vi "header.vi"(0 "Signals":dbl[](array[numeric]), 2 "标准差 V":dbl=0.02 format="%.2p", 3 "采样数 k":dbl=3000.0, 4 "Lower Cut-Off":dbl=280000.0, 8 "采样率 MHz":dbl=50.0, 9 "f_c kHz":dbl=150.0, 10 "A_c V":dbl=1.0, 11 "k_f kHz/V":dbl=50.0) -> (5 "解调复原的基带信号":waveform(dbl)(graph), 6 "已调信号频域波形观测":dynamicdata(graph), 7 "信号时域波形观测":dynamicdata(graph))   [LabVIEW 2020]
uses:
  <vilib>/express/express shared/transition.llb/Dynamic To Waveform Array.vi
  <vilib>/express/express arith-compare/Formula/Block/exnFormulaBlock how many pts in the wave.vi
  <vilib>/express/express shared/ex_Modify Signal Name.vi
  <vilib>/express/express shared/transition.llb/Waveform Array To Dynamic.vi
  <vilib>/express/express analysis/Spectral/Block/exnSpectralBlock spectral measurements peak poly.vi
  <vilib>/express/express analysis/Spectral/Block/exnSpectralBlock spectral measurements peak DDT.vi
  <vilib>/express/express arith-compare/Formula/XNode/ExpressFormulaBlockNode.xnode
  <vilib>/express/express analysis/Spectral/XNode/ExpressSpectralMeasurementsBlockNode.xnode
  <vilib>/measure/NI_MABase.lvlib
  <vilib>/Analysis/NI_AALPro.lvlib
panel:
  out "f_c Hz":dbl
  out "采样数":dbl
  out "采样率 Hz":dbl
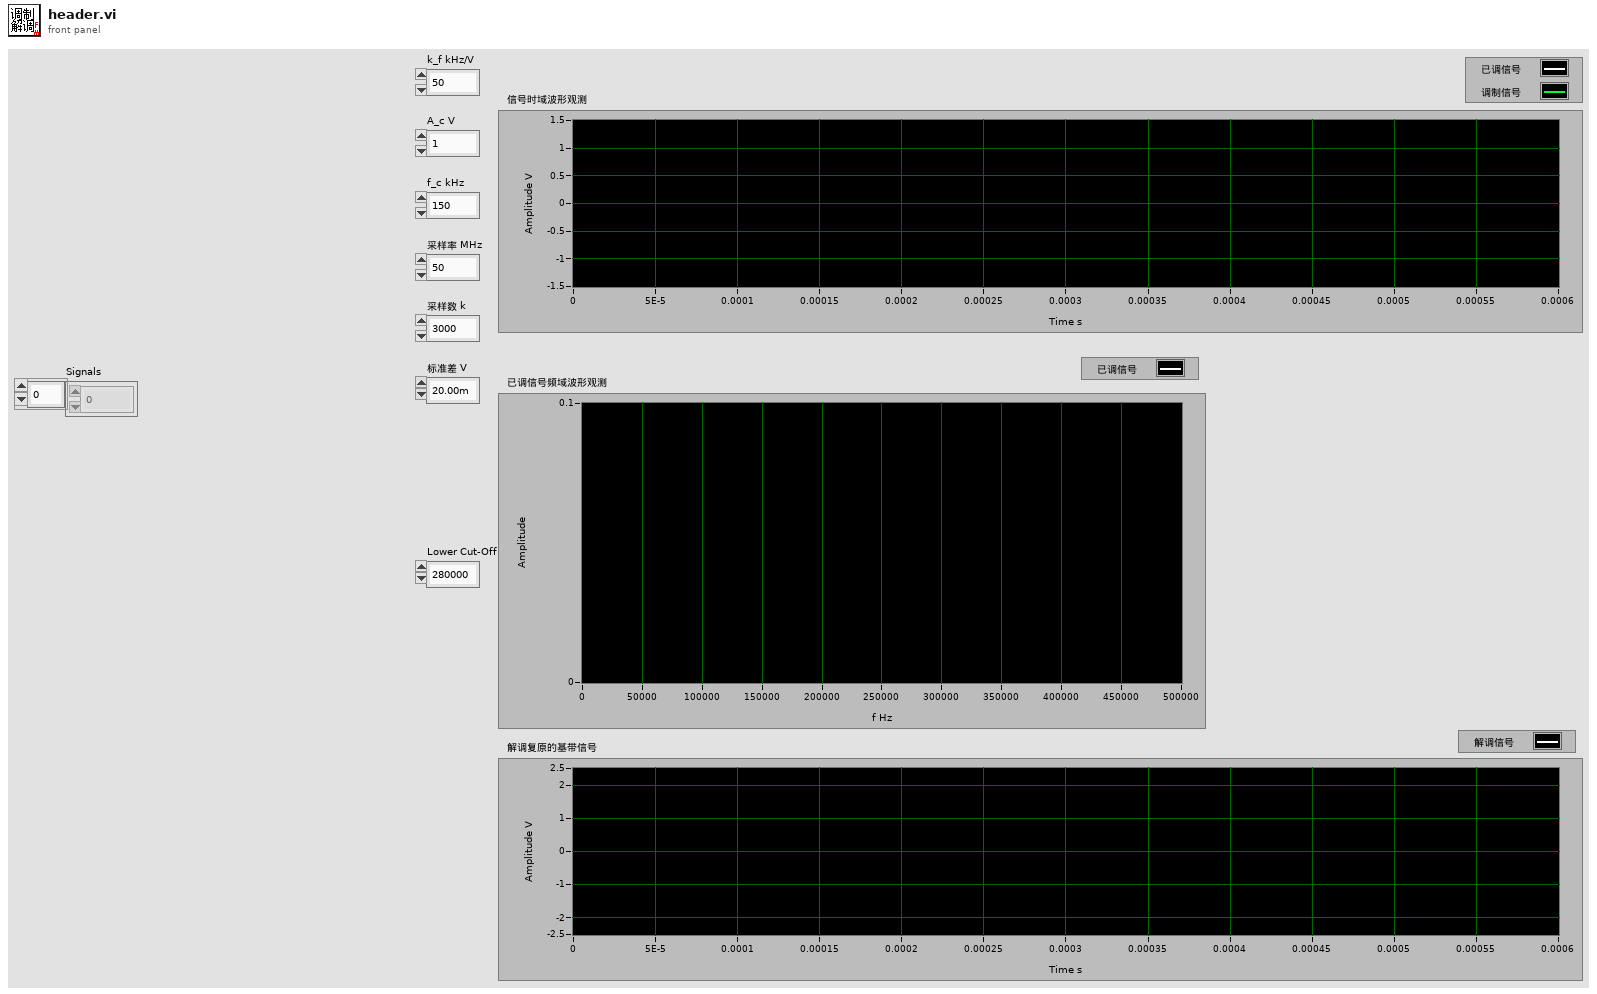
[diagram p1: front panel]
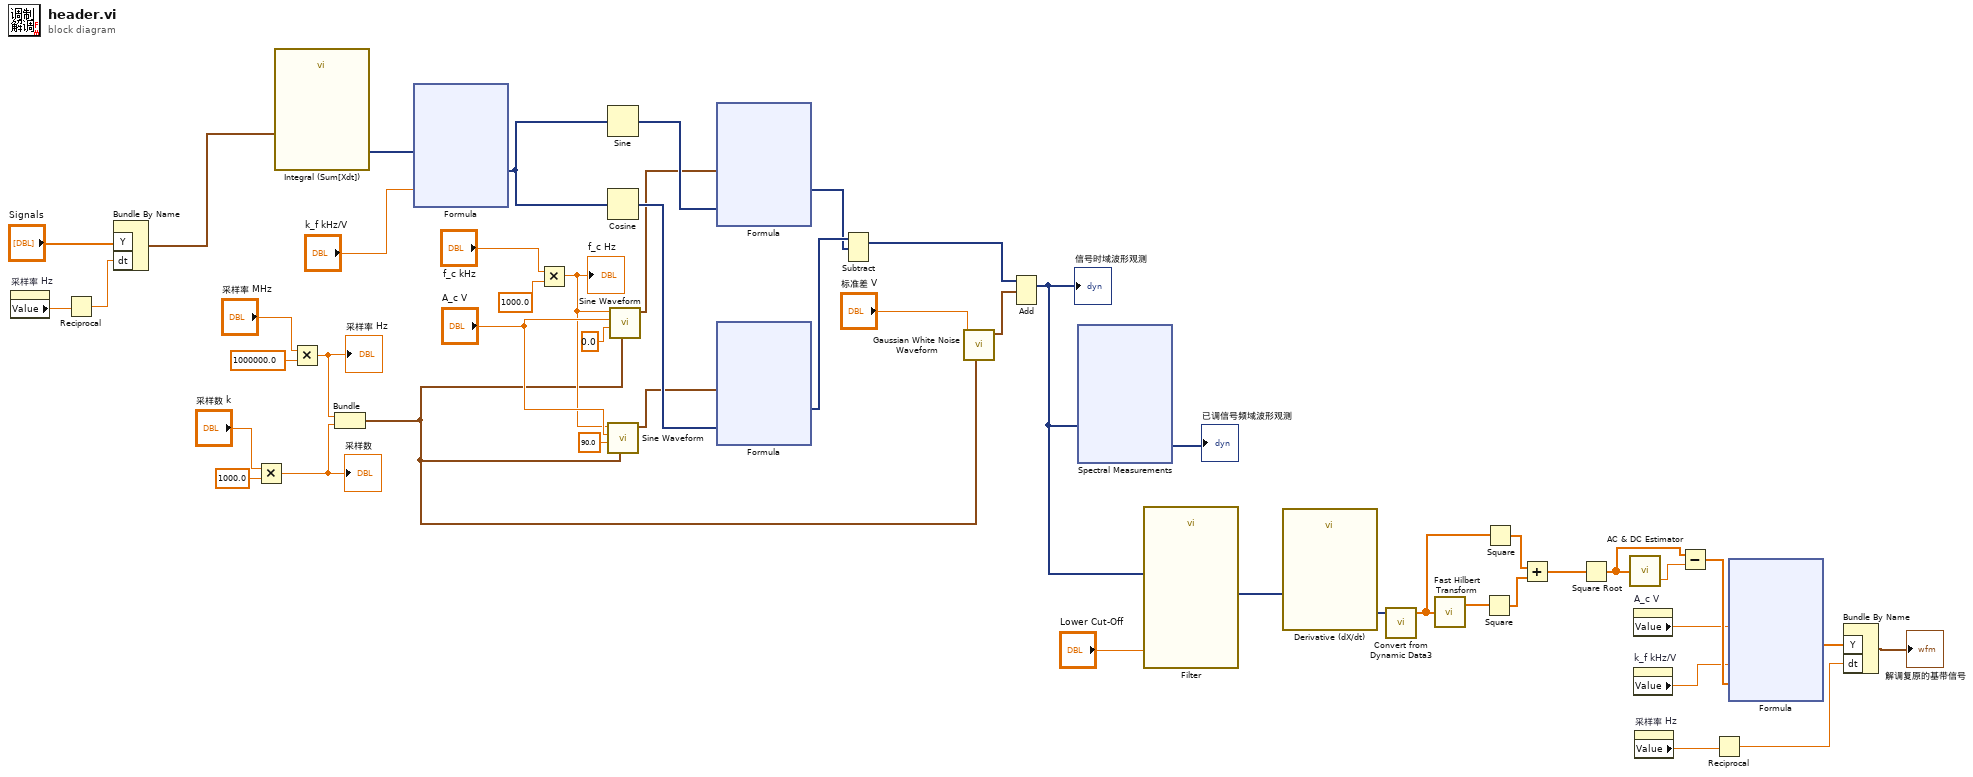
[diagram p0: block diagram]
diagram:
  n1 = property on="采样率 Hz" class="DigNum (strict)"() -> ("Value"=w2:dbl)  [unwired: 2 in, 2 out]
  n2 = Reciprocal(x=w2) -> (1/x=w5:dbl)
  n3 = Bundle By Name("Y"="Signals", "dt"=w5) -> (w3:waveform(dbl))  [unwired: 1 in]
  n4 = Multiply(x="采样数 k", y=1000.0) -> (x*y=w35:dbl)
  "采样数" <- w35
  n5 = call "Integral (Sum[Xdt])"("Signals"=w3) -> ("Result"=w25:dynamicdata)  [unwired: 5 in, 1 out]
  n6 = Multiply(x="采样率 MHz", y=1000000.0) -> (x*y=w38:dbl)
  "采样率 Hz" <- w38
  n7 = Bundle(w38, w35) -> (w23:cluster{dbl, dbl})  [unwired: 1 in]
  n8 = xnode "Formula"("积分后的信号"=w25, "k_f"="k_f kHz/V") -> ("Result"=w47:dynamicdata)  [unwired: 1 in, 1 out]
  n9 = Multiply(x="f_c kHz", y=1000.0) -> (x*y=w41:dbl)
  "f_c Hz" <- w41
  n10 = Sine(x=w47) -> (sin(x)=w33:dynamicdata)
  n11 = Cosine(x=w47) -> (cos(x)=w34:dynamicdata)
  n12 = call <vilib>:"Sine Waveform.vi"("sampling info"=w23, "phase"=90.0, "amplitude"="A_c V", "frequency"=w41) -> ("signal out"=w31:waveform(dbl))  [unwired: 6 in, 1 out]
  n13 = call <vilib>:"Sine Waveform.vi"("sampling info"=w23, "phase"=0.0, "amplitude"="A_c V", "frequency"=w41) -> ("signal out"=w32:waveform(dbl))  [unwired: 6 in, 1 out]
  n14 = xnode "Formula"("sin载波"=w32, "sin相偏"=w33) -> ("Result"=w29:dynamicdata)  [unwired: 1 in, 1 out]
  n15 = xnode "Formula"("cos载波"=w31, "cos相偏"=w34) -> ("Result"=w30:dynamicdata)  [unwired: 1 in, 1 out]
  n16 = Subtract(1:w29, 2:w30) -> (0:w27:dynamicdata)  [unwired: 1 in, 1 out]
  n17 = call <vilib>:"Gaussian White Noise Waveform.vi"("sampling info"=w23, "standard deviation"="标准差 V") -> ("signal out"=w26:waveform(dbl))  [unwired: 8 in, 1 out]
  n18 = Add(1:w26, 2:w27) -> (0:w1:dynamicdata)  [unwired: 1 in, 1 out]
  "信号时域波形观测" <- w1
  n19 = xnode "Spectral Measurements"("Signals"=w1) -> ("FFT - (Peak)"=→"已调信号频域波形观测":dynamicdata)  [unwired: 1 in, 2 out]
  n20 = call "Filter"("Lower Cut-Off"="Lower Cut-Off", "Signal"=w1) -> ("Filtered Signal"=w7:dynamicdata)  [unwired: 8 in, 1 out]
  n21 = call "Derivative (dX/dt)"("Signals"=w7) -> ("Result"=w17:dynamicdata)  [unwired: 5 in, 1 out]
  n22 = call "Convert from Dynamic Data3"("Dynamic Data Type"=w17) -> ("Array"=w22:dbl[])  [unwired: 3 in]
  n23 = call <vilib>:"Fast Hilbert Transform.vi"("X"=w22) -> ("Hilbert{X}"=w21:dbl[])  [unwired: 1 out]
  n24 = Square(x=w21) -> (x^2=w19:dbl[])
  n25 = Square(x=w22) -> (x^2=w20:dbl[])
  n26 = Add(x=w20, y=w19) -> (x+y=w18:dbl[])
  n27 = Square Root(x=w18) -> (sqrt(x)=w16:dbl[])
  n28 = call <vilib>:"AC & DC Estimator.vi"("Signal (V)"=w16) -> ("DC estimate (V)"=w12:dbl)  [unwired: 1 out]
  n29 = property on="A_c V" class="DigNum (strict)"() -> ("Value"=w10:dbl)  [unwired: 2 in, 2 out]
  n30 = property on="k_f kHz/V" class="DigNum (strict)"() -> ("Value"=w9:dbl)  [unwired: 2 in, 2 out]
  n31 = property on="采样率 Hz" class="DigNum (strict)"() -> ("Value"=w15:dbl)  [unwired: 2 in, 2 out]
  n32 = Subtract(x=w16, y=w12) -> (x-y=w11:dbl[])
  n33 = Reciprocal(x=w15) -> (1/x=w14:dbl)
  n34 = xnode "Formula"("A_c"=w10, "k_f"=w9, "Signals"=w11) -> ("Result"=w8:dbl[])  [unwired: 1 in, 1 out]
  n35 = Bundle By Name("Y"=w8, "dt"=w14) -> (→"解调复原的基带信号":waveform(dbl))  [unwired: 1 in]
